vi "GetText.vi"(8 "error in":errorcluster, 11 "SequenceNode in":refnum<class "SequenceNode.lvclass">) -> (0 "error out":errorcluster, 1 "additional text":string, 2 "text":string, 3 "SequenceNode out":refnum<class "SequenceNode.lvclass">, 4 "glyph":string)   [LabVIEW 2015, in "SequenceNode.lvclass"]
doc: "Copyright 2017 National Instruments Corporation\n\nLicensed under the Apache License, Version 2.0 (the \"License\"); you may not use this file except in compliance with the License. You may obtain a copy of the License at http://www.apache.org/licenses/LICENSE-2.0\nUnless required by applicable law or agreed to in writing, software distributed under the License is distributed on an \"AS IS\" BASIS, WITHOUT WARRANTIES OR CONDITIONS OF ANY KIND, either express or implied. See the License for the specific language governing permissions and limitations under the License."
uses:
  SequenceNode.lvclass
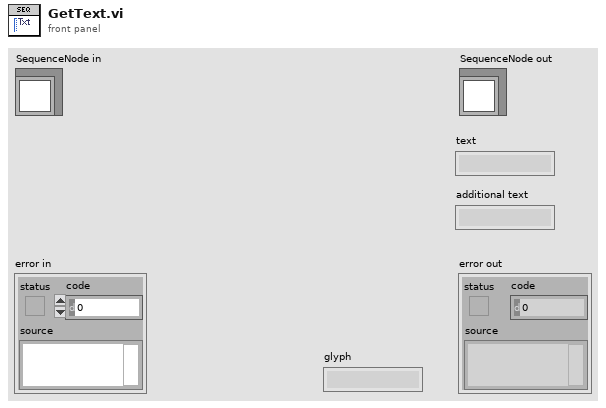
[diagram p1: front panel]
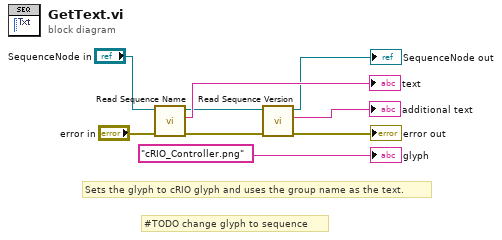
[diagram p0: block diagram]
diagram:
  # "#TODO change glyph to sequence"
  # "Sets the glyph to cRIO glyph and uses the group name as the text."
  n1 = call-dynamic "Read Sequence Name.vi"("error in (no error)"="error in", "SequenceNode in"="SequenceNode in") -> ("error out"=w7:errorcluster, "Sequence Name"=→"text":string, "SequenceNode out"=w3:refnum<class "SequenceNode.lvclass">)  [unwired: 7 in]
  n2 = call-dynamic "Read Sequence Version.vi"("error in (no error)"=w7, "SequenceNode in"=w3) -> ("error out"=→"error out":errorcluster, "Sequence Version"=→"additional text":string, "SequenceNode out"=→"SequenceNode out":refnum<class "SequenceNode.lvclass">)  [unwired: 7 in]
  "glyph" <- "cRIO_Controller.png" ("glyph")
